vi "BeltControlOverhaul.vi"(4 "Roll Out":bool, 5 "Top Eye":bool, 6 "Intake":bool, 7 "Score":bool, 8 "Lower Eye":bool, 9 "Middle Eye":bool) -> (0 "Sidways Motor":T1, 1 "Lower Motor":i32=1, 2 "Middle Motor":i32=1, 3 "Top Motor":i32=1)   [LabVIEW 2011]
doc: "A subVI handling the whole intake system, from the drop-down extension to the shooter feeding rollers."
uses:
  <vilib>/Rock Robotics/WPI/Relay/WPI_RelayValue.ctl
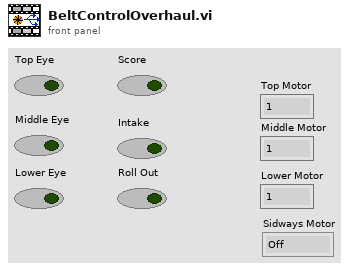
[diagram p1: front panel]
types:
  T1 = typedef "WPI_RelayValue.ctl" = enum16{"Off", "On", "Forward", "Reverse"}
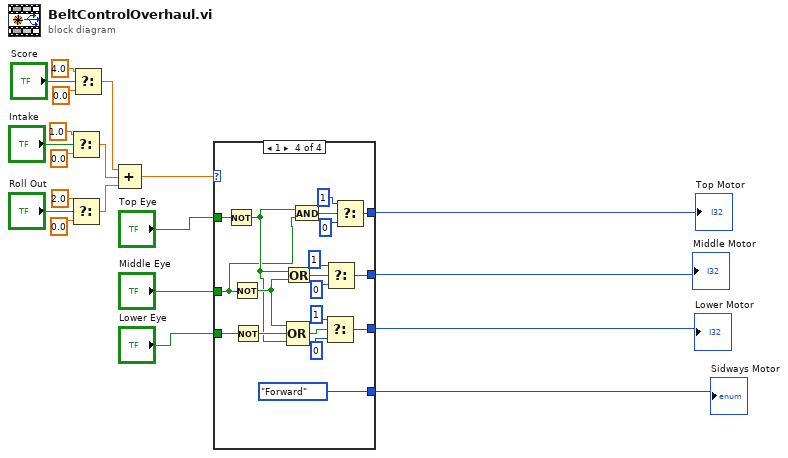
[diagram p0: block diagram]
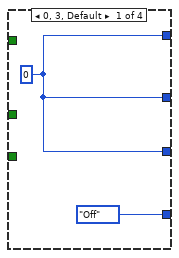
[diagram p2: hidden frame]
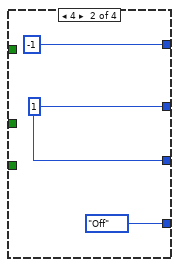
[diagram p3: hidden frame]
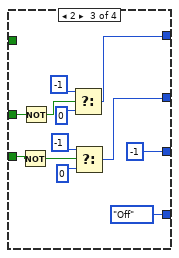
[diagram p4: hidden frame]
diagram:
  n1 = Select(t=1.0, s="Intake", f=0.0 ("t")) -> (s? t:f=w6:dbl)
  n2 = Select(t=2.0, s="Roll Out", f=0.0 ("t")) -> (s? t:f=w7:dbl)
  n3 = Select(t=4.0, s="Score", f=0.0 ("t")) -> (s? t:f=w5:dbl)
  n4 = Compound Arithmetic op=ADD(w5, w6, w7) -> (w8:dbl)
  n5 = case shown="1" w8 {
    tunnel: [w22 -1 ("f") w34 w41] -> w20
    tunnel: [w22 w24 w35 w53] -> w19
    tunnel: [w22 w24 -1 ("f") w50] -> w18
    tunnel: "Top Eye" -> [_ _ _ w48]
    tunnel: "Middle Eye" -> [_ _ w29 w38]
    tunnel: "Lower Eye" -> [_ _ w26 w47]
    tunnel: [WPI_RelayValue."Off" ("RelayValue") WPI_RelayValue."Off" ("RelayValue") WPI_RelayValue."Off" ("RelayValue") WPI_RelayValue."Forward" ("RelayValue")] -> w4
    frame 0, 3, Default {
      w22 = 0
    }
    frame 4 {
      w24 = 1 ("f")
    }
    frame 2 {
      n6 = Not(x=w26) -> (.not. x?=w27:bool)
      n7 = Not(x=w29) -> (.not. x?=w28:bool)
      n8 = Select(t=-1 ("f"), s=w28, f=0) -> (s? t:f=w34:i32)
      n9 = Select(t=-1 ("f"), s=w27, f=0) -> (s? t:f=w35:i32)
    }
    frame 1 {
      n10 = Not(x=w48) -> (.not. x?=w39:bool)
      n11 = Not(x=w38) -> (.not. x?=w45:bool)
      n12 = Not(x=w47) -> (.not. x?=w44:bool)
      n13 = Or(x=w39, y=w45) -> (x .or. y?=w54:bool)
      n14 = Compound Arithmetic op=OR(w45, w44, w39) -> (w46:bool)
      n15 = And(x=w39, y=w38) -> (x .and. y?=w40:bool)
      n16 = Select(t=i8 1, s=w46, f=i8 0) -> (s? t:f=w50:i8)
      n17 = Select(t=i8 1, s=w54, f=i8 0) -> (s? t:f=w53:i8)
      n18 = Select(t=i8 1, s=w40, f=i8 0) -> (s? t:f=w41:i8)
    }
  }
  "Top Motor" <- w20
  "Middle Motor" <- w19
  "Lower Motor" <- w18
  "Sidways Motor" <- w4
